vi "Json_Specific part.vi"(8 "error in (no error)":errorcluster, 9 "Zen Analytics in":refnum<class "Zen Analytics.lvclass">, 10 "JSON Cluster":T2, 11 "Part-num":string) -> (0 "error out":errorcluster, 3 "Json Part no specicific op":T1)   [LabVIEW 2019, in "Zen Analytics.lvlib" / "Zen Analytics.lvclass"]
uses:
  Zen Analytics.lvclass
  Dependency/Json Partno Specific output.ctl
  Dependency/GraphReff.ctl
  <vilib>/ActorFramework/Message Enqueuer/Message Enqueuer.lvclass
  Dependency/AnalyticsDataToSM.ctl
  Dependency/JSON Cluster(Int).ctl
types:
  T1 = typedef "Zen Analytics.lvlib/Zen Analytics.lvclass/Json Partno Specific output.ctl" = cluster{"Array Params ":cluster{"RowsIn2DArray":i32, "ColumnsIn2DArray":i32, "SamplesToDisplay":i32, "UpdateRate":string}, "PlotParameters":cluster{"Trend":cluster{"TrendPlotID":dbl, "PlotProperties":cluster{"FontName":string, "FontSize":dbl, "FontColor":string, "IsBold":bool, "IsItalic":bool, "PlotColor":string}}[], "Histogram":cluster{"HistogramPlotID":dbl, "PlotProperties":cluster{"FontName":string, "FontSize":dbl, "FontColor":string, "IsBold":bool, "IsItalic":bool, "PlotColor":string}}[], "BarPlot":cluster{"BarPlotID":dbl, "BarValuesID":dbl, "PlotProperties":cluster{"FontName":string, "FontSize":dbl, "IsBold":bool, "IsItalic":bool, "FontColor":string}, "Sectors":string[]}[], "PieChart":cluster{"PieChartID":dbl, "PieChartValueID":dbl, "PlotProperties":cluster{"FontName":string, "FontSize":dbl, "IsBold":bool, "IsItalic":bool, "FontColor":string}, "Sectors":string[]}[]}}
  T2 = typedef "Zen Analytics.lvlib/Zen Analytics.lvclass/JSON Cluster(Int).ctl" = cluster{"Rows In 2D Array":i32, "Columns In 2D Array":i32, "Samples To Display":i32, "Update Rate (Time)":i32, "Update Rate (Samples)":i32, "CurrentPartNumber":string, "AnalyticsDataFormat":cluster{"AnalyticsParameters":cluster{"UpdateRateCategories":cluster{"LOW":cluster{"SampleElapsed":dbl, "TimeElapsed":dbl}, "MEDIUM":cluster{"SampleElapsed":dbl, "TimeElapsed":dbl}, "HIGH":cluster{"SampleElapsed":dbl, "TimeElapsed":dbl}}, "AnalyticsForPartsList":cluster{"Name":string, "InitializationValues":cluster{"RowsIn2DArray":dbl, "ColumnsIn2DArray":dbl, "SamplesToDisplay":dbl, "UpdateRate":string}, "PlotParameters":cluster{"Trend":cluster{"TrendPlotID":dbl, "PlotProperties":cluster{"FontName":string, "FontSize":dbl, "FontColor":string, "IsBold":bool, "IsItalic":bool, "PlotColor":string}}[], "Histogram":cluster{"HistogramPlotID":dbl, "PlotProperties":cluster{"FontName":string, "FontSize":dbl, "FontColor":string, "IsBold":bool, "IsItalic":bool, "PlotColor":string}}[], "BarPlot":cluster{"BarPlotID":dbl, "BarValuesID":dbl, "PlotProperties":cluster{"FontName":string, "FontSize":dbl, "IsBold":bool, "IsItalic":bool, "FontColor":string}, "Sectors":string[]}[], "PieChart":cluster{"PieChartID":dbl, "PieChartValueID":dbl, "PlotProperties":cluster{"FontName":string, "FontSize":dbl, "IsBold":bool, "IsItalic":bool, "FontColor":string}, "Sectors":string[]}[]}}[]}}, "MeasurementData":cluster{"Measurement ID":i32, "Measurement Name":string, "Nominal Values":dbl, "LSL":dbl, "USL":dbl, "LCL":dbl, "UCL":dbl}[], "PlotParameters":cluster{"Trend":cluster{"TrendPlotID":dbl, "PlotProperties":cluster{"FontName":string, "FontSize":dbl, "FontColor":string, "IsBold":bool, "IsItalic":bool, "PlotColor":string}}[], "Histogram":cluster{"HistogramPlotID":dbl, "PlotProperties":cluster{"FontName":string, "FontSize":dbl, "FontColor":string, "IsBold":bool, "IsItalic":bool, "PlotColor":string}}[], "BarPlot":cluster{"BarPlotID":dbl, "BarValuesID":dbl, "PlotProperties":cluster{"FontName":string, "FontSize":dbl, "IsBold":bool, "IsItalic":bool, "FontColor":string}, "Sectors":string[]}[], "PieChart":cluster{"PieChartID":dbl, "PieChartValueID":dbl, "PlotProperties":cluster{"FontName":string, "FontSize":dbl, "IsBold":bool, "IsItalic":bool, "FontColor":string}, "Sectors":string[]}[]}}
  T3 = typedef "Zen Analytics.lvlib/Zen Analytics.lvclass/AnalyticsDataToSM.ctl" = cluster{"Actor Info":cluster{"Analytics Enqueuer":refnum<class "Message Enqueuer.lvclass">, "This VI":refnum<vi>, "Module name":string}, "Statistical Info":string[][], "Graph Refference's":T4, "ErrorMessage":string}
  T4 = typedef "Zen Analytics.lvlib/Zen Analytics.lvclass/GraphReff.ctl" = cluster{"HistgramGraph-reff":refnum<vi>[], "BarGraph-reff":refnum<vi>[], "PieGraph-reff":refnum<vi>[], "Lable-reff":refnum<vi>[], "TrendGraph-reff":refnum<vi>[], "CpCpkTable":refnum<vi>}
  T5 = cluster{"Name":string, "InitializationValues":cluster{"RowsIn2DArray":dbl, "ColumnsIn2DArray":dbl, "SamplesToDisplay":dbl, "UpdateRate":string}, "PlotParameters":cluster{"Trend":cluster{"TrendPlotID":dbl, "PlotProperties":cluster{"FontName":string, "FontSize":dbl, "FontColor":string, "IsBold":bool, "IsItalic":bool, "PlotColor":string}}[], "Histogram":cluster{"HistogramPlotID":dbl, "PlotProperties":cluster{"FontName":string, "FontSize":dbl, "FontColor":string, "IsBold":bool, "IsItalic":bool, "PlotColor":string}}[], "BarPlot":cluster{"BarPlotID":dbl, "BarValuesID":dbl, "PlotProperties":cluster{"FontName":string, "FontSize":dbl, "IsBold":bool, "IsItalic":bool, "FontColor":string}, "Sectors":string[]}[], "PieChart":cluster{"PieChartID":dbl, "PieChartValueID":dbl, "PlotProperties":cluster{"FontName":string, "FontSize":dbl, "IsBold":bool, "IsItalic":bool, "FontColor":string}, "Sectors":string[]}[]}}[]
  T6 = cluster{"RowsIn2DArray":dbl, "ColumnsIn2DArray":dbl, "SamplesToDisplay":dbl, "UpdateRate":string}
  T7 = cluster{"Trend":cluster{"TrendPlotID":dbl, "PlotProperties":cluster{"FontName":string, "FontSize":dbl, "FontColor":string, "IsBold":bool, "IsItalic":bool, "PlotColor":string}}[], "Histogram":cluster{"HistogramPlotID":dbl, "PlotProperties":cluster{"FontName":string, "FontSize":dbl, "FontColor":string, "IsBold":bool, "IsItalic":bool, "PlotColor":string}}[], "BarPlot":cluster{"BarPlotID":dbl, "BarValuesID":dbl, "PlotProperties":cluster{"FontName":string, "FontSize":dbl, "IsBold":bool, "IsItalic":bool, "FontColor":string}, "Sectors":string[]}[], "PieChart":cluster{"PieChartID":dbl, "PieChartValueID":dbl, "PlotProperties":cluster{"FontName":string, "FontSize":dbl, "IsBold":bool, "IsItalic":bool, "FontColor":string}, "Sectors":string[]}[]}
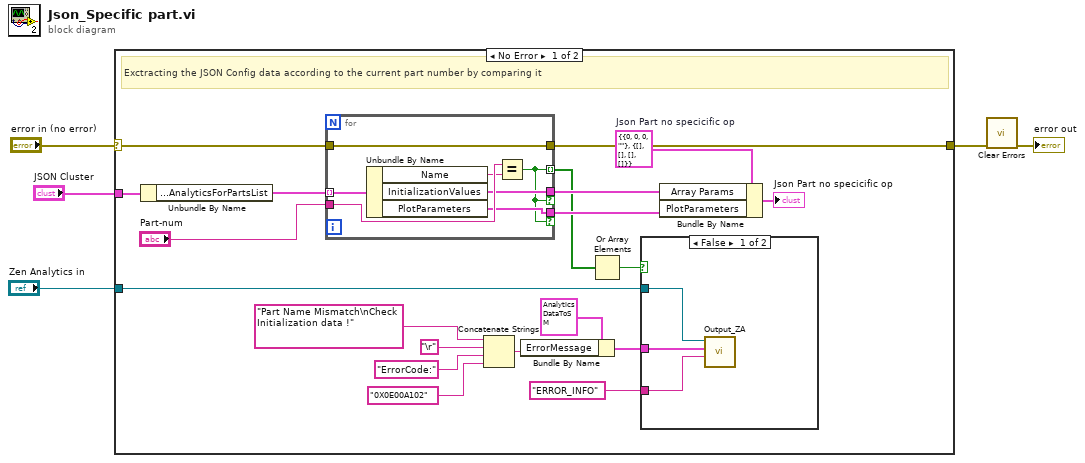
[diagram p0: block diagram]
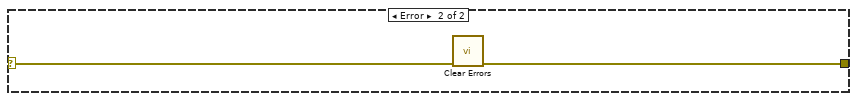
[diagram p3: hidden frame]
diagram:
  n1 = case shown="No Error" "error in (no error)" {
    selector: "error in (no error)" -> [w24 w37]
    tunnel: [w23 w36] -> w2
    tunnel: "JSON Cluster" -> [w22 _]
    tunnel: "Zen Analytics in" -> [w6 _]
    frame No Error {
      w20 = T1 {"Array Params "={"RowsIn2DArray"=0, "ColumnsIn2DArray"=0, "SamplesToDisplay"=0, "UpdateRate"=""}, "PlotParameters"={"Trend"=[], "Histogram"=[], "BarPlot"=[], "PieChart"=[]}}  # Json Part no specicific op
      # "Exctracting the JSON Config data according to the current part number by comparing it"
      n2 = Unbundle By Name(w22) -> ("AnalyticsDataFormat.AnalyticsParameters.AnalyticsForPartsList"=w21:T5)
      n3 = for {
        tunnel: w21 -> [w33] mode=indexing
        tunnel: "Part-num" -> [w34]
        tunnel: [w31] -> w19 if=w29
        tunnel: [w30] -> w18 if=w29
        tunnel: w24 -> [w35]
        tunnel: [w35] -> w23
        tunnel: [w29] -> w16 mode=indexing
        n4 = Unbundle By Name(w33) -> ("Name"=w32:string, "InitializationValues"=w31:T6, "PlotParameters"=w30:T7)
        n5 = Equal?(x=w34, y=w32) -> (x = y?=w29:bool)
      }
      n6 = Concatenate Strings("Part Name Mismatch\nCheck Initialization data !" ("SolutionForError"), "\r", "ErrorCode:", "0X0E00A102" ("ErrorCode")) -> (w9:string)
      n7 = Bundle By Name(cluster=T3 {"Actor Info"={"Analytics Enqueuer"=refnum, "This VI"=refnum, "Module name"=""}, "Statistical Info"=[], "Graph Refference's"={"HistgramGraph-reff"=[], "BarGraph-reff"=[], "PieGraph-reff"=[], "Lable-reff"=[], "TrendGraph-reff"=[], "CpCpkTable"=refnum}, "ErrorMessage"=""} ("Analytics Information"), "ErrorMessage"=w9) -> (w8:T3)
      n8 = Or Array Elements(Boolean array=w16) -> (logical OR=w15:bool)
      n9 = case shown="False" w15 {
        tunnel: w8 -> [w28 _]
        tunnel: "ERROR_INFO" ("State") -> [w27 _]
        tunnel: w6 -> [w26 _]
        frame False {
          n10 = call "Output_ZA.vi"("State"=w27, "Analytics Information"=w28, "Zen Analytics in"=w26) -> ()  [unwired: 7 in, 2 out]
        }
        frame True {
        }
      }
      n11 = Bundle By Name(cluster=w20, "Array Params"=w19, "PlotParameters"=w18) -> (→"Json Part no specicific op":T1)
    }
    frame Error {
      n12 = call <vilib>:"Clear Errors.vi"("error in (no error)"=w37) -> ("error out"=w36:errorcluster)  [unwired: 5 in, 1 out]
    }
  }
  n13 = call <vilib>:"Clear Errors.vi"("error in (no error)"=w2) -> ("error out"=→"error out":errorcluster)  [unwired: 5 in, 1 out]
